vi "Output_single_waveform.vi"() -> ()   [LabVIEW 2015]
uses:
  Create_waveform/build_waveform.lvclass
  Write_to_file/Write_to_file.lvclass
  Plot_waveform/Plot_waveform.lvclass
panel:
  out "Waveform":waveform(dbl)(graph)={"t0"=timestamp(0 s since 1904-01-01), "dt"=8.333333333333334e-10, "Y"=array[8192 elements]}
  in  "start path":path=path "C:/GitHub/PulseEcho/PulsedFieldEcho/Create_Pulse"
  in  "standard deviation":dbl=0.1
  in  "NWaves":i32=10
  in  "Frequency":dbl=220000000.0
  in  "clock rate":dbl=1200000000.0
  # "Select Path"
  # "Pulse Parameters"
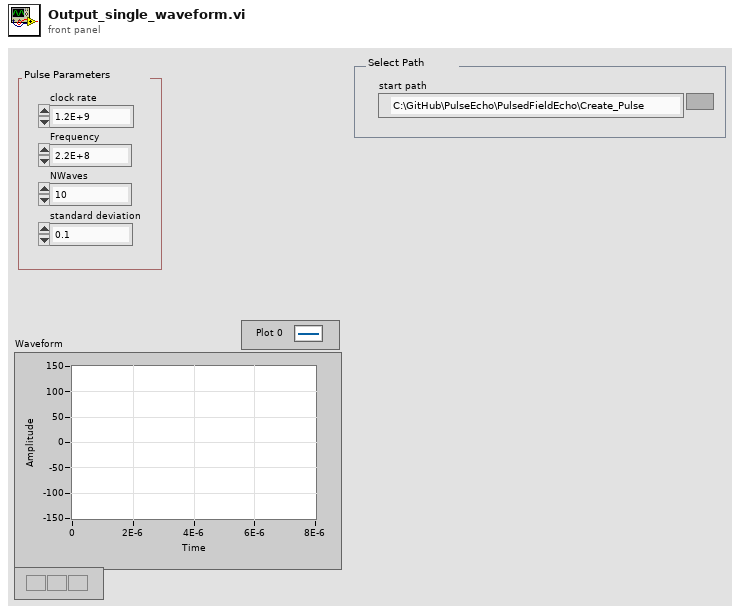
[diagram p1: front panel]
types:
  T1 = enum16{"open", "replace", "create", "open or create", "replace or create", "replace or create with confirmation"}
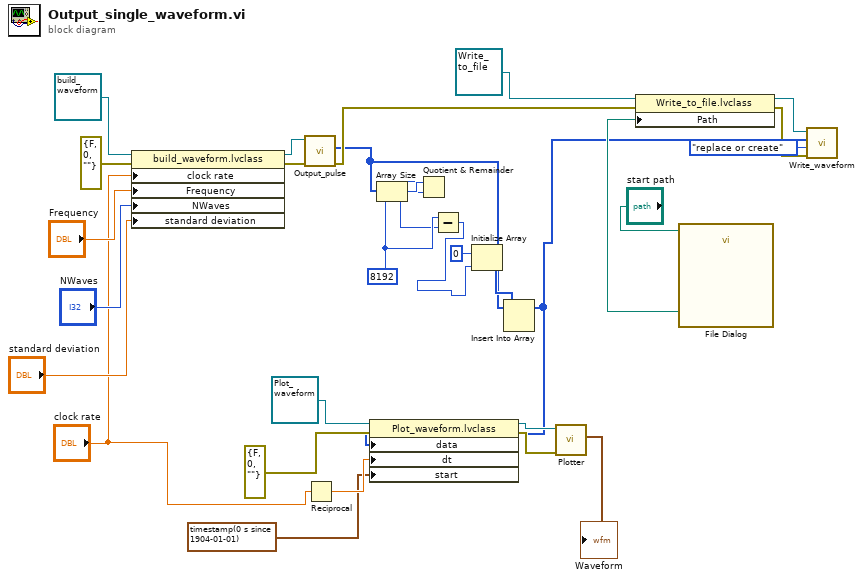
[diagram p0: block diagram]
diagram:
  w7 = 8192
  n1 = property class="build_waveform.lvclass"(reference=refnum<class "build_waveform.lvclass"> refnum ("build_waveform.lvclass"), error in=errorcluster {"status"=FALSE, "code"=0, "source"=""} ("error in (no error)"), "clock rate"="clock rate", "Frequency"="Frequency", "NWaves"="NWaves", "standard deviation"="standard deviation") -> (reference out=w25:refnum<class "build_waveform.lvclass">, error out=w24:errorcluster)
  n2 = call-dynamic "Output_pulse.vi"("error in (no error)"=w24, "build_waveform in"=w25) -> ("error out"=w10:errorcluster, "Array"=w2:i8[])  [unwired: 7 in, 1 out]
  n3 = Reciprocal(x="clock rate") -> (1/x=w19:dbl)
  n4 = Array Size(array=w2) -> (size(s)=w8:i32)
  n5 = Quotient & Remainder(x=w8, y=w7) -> (x-y*floor(x/y)=w6:i32)  [unwired: 1 out]
  n6 = Subtract(x=w7, y=w6) -> (x-y=w3:i32)
  n7 = Initialize Array(i16 0 ("element"), w3) -> (w4:i16[])
  n8 = Insert Into Array(array=w2, new element=w4) -> (w1:i8[])  [unwired: 1 in]
  n9 = property class="Plot_waveform.lvclass"(reference=refnum<class "Plot_waveform.lvclass"> refnum ("Plot_waveform.lvclass"), error in=errorcluster {"status"=FALSE, "code"=0, "source"=""} ("error in (no error)"), "data"=w1, "dt"=w19, "start"=timestamp(0 s since 1904-01-01)) -> (reference out=w17:refnum<class "Plot_waveform.lvclass">, error out=w16:errorcluster)
  n10 = call-dynamic "Plotter.vi"("error in (no error)"=w16, "Plot_waveform in"=w17) -> ("output waveform"=→"Waveform":waveform(dbl))  [unwired: 7 in, 2 out]
  n11 = call "File Dialog"("start path"="start path") -> ("selected path"=w23:path)  [unwired: 11 in, 3 out]
  n12 = property class="Write_to_file.lvclass"(reference=refnum<class "Write_to_file.lvclass"> refnum ("Write_to_file.lvclass"), error in=w10, "Path"=w23) -> (reference out=w11:refnum<class "Write_to_file.lvclass">, error out=w13:errorcluster)
  n13 = call-dynamic "Write_waveform.vi"("error in (no error)"=w13, "operation (0:open)"=T1."replace or create", "Array"=w1, "Write_to_file in"=w11) -> ()  [unwired: 6 in, 2 out]
